vi "Strip Extensions from Qualified Name.vi"(10 "Qualified Name":string) -> (2 "Qualified Name without File Extensions":string)   [LabVIEW 2020]
doc: "Strip the file extensions from the qualified name string. So \"a.lvlib:b.lvlib:c.lvclass\" becomes \"a:b:c\"."
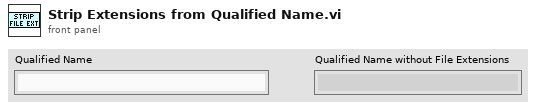
[diagram p1: front panel]
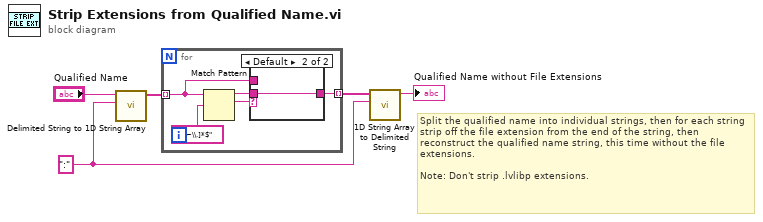
[diagram p0: block diagram]
diagram:
  w1 = ":" ("delimiter")
  # "Split the qualified name into individual strings, then for each string strip off the file extension from the end of the string, then reconstruct the qualified name string, this time without the file extensions.\n\nNote: Don't strip .lvlibp extensions."
  n1 = call <vilib>:"Delimited String to 1D String Array.vi"("delimiter"=w1, "delimited string"="Qualified Name") -> ("string array"=w4:string[])  [unwired: 9 in]
  n2 = for {
    tunnel: w4 -> [w6] mode=indexing
    tunnel: [w8] -> w3 mode=indexing
    n3 = Match Pattern(string=w6, regular expression="\\.[~\\.]*$") -> (before substring=w7:string, match substring=w9:string)  [unwired: 3 out]
    n4 = case shown="Default" w9 {
      tunnel: [w11 w12] -> w8
      tunnel: w7 -> [_ w12]
      tunnel: w6 -> [w11 _]
      frame ".lvlibp" {
      }
      frame Default {
      }
    }
  }
  n5 = call <vilib>:"1D String Array to Delimited String.vi"("delimiter"=w1, "string array"=w3) -> ("delimited string"=→"Qualified Name without File Extensions":string)  [unwired: 9 in]
